vi "Generate Unique Header.vi"(8 "error in":errorcluster, 11 "mTEC Data in":refnum<class "mTEC Data.lvclass">) -> (0 "error out":errorcluster, 2 "Header":string[](array[string]), 3 "mTEC Data out":refnum<class "mTEC Data.lvclass">)   [LabVIEW 2014, in "Meerstetter Lib.lvlib" / "mTEC Data.lvclass"]
uses:
  mTEC Data.lvclass
  reusable/Data/Data.lvclass/Data.ctl
  reusable/Data/Read Data ID.vi
  reusable/Data/Data.lvclass
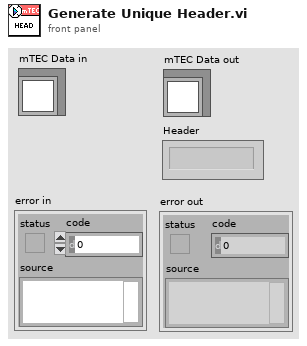
[diagram p1: front panel]
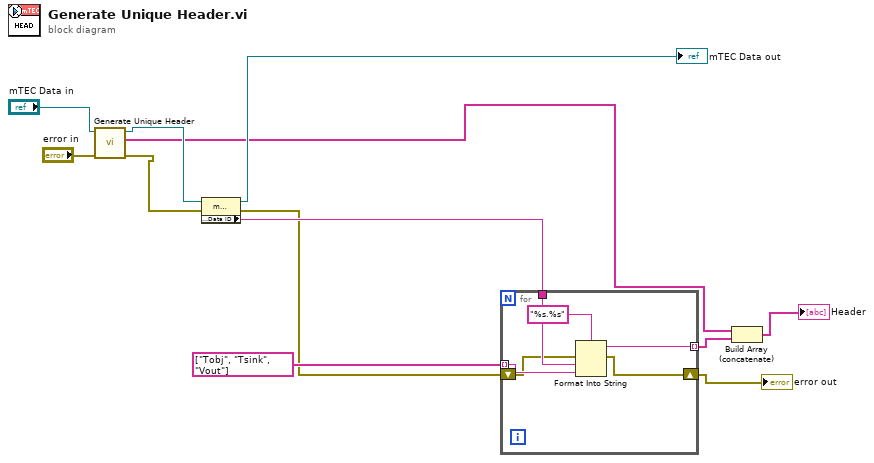
[diagram p0: block diagram]
diagram:
  n1 = call-parent "Generate Unique Header.vi"("error in"="error in", "Data in"="mTEC Data in") -> ("error out"=w8:errorcluster, "Header"=w2:string[], "Data out"=w9:refnum<class "mTEC Data.lvclass">)  [unwired: 7 in]
  n2 = property class="mTEC Data.lvclass"(reference=w9, error in=w8) -> (reference out=→"mTEC Data out":refnum<class "mTEC Data.lvclass">, error out=w6:errorcluster, "Accessors:Data ID"=w7:string)
  n3 = for {
    tunnel: string[] ["Tobj", "Tsink", "Vout"] -> [w17] mode=indexing
    tunnel: w7 -> [w18]
    tunnel: [w15] -> w3 mode=indexing
    shift-right: [w14] -> w4
    shift-left: w6 -> [w13]
    n4 = Format Into String(format string="%s.%s", error in=w13, w18, w17) -> (resulting string=w15:string, error out=w14:errorcluster)  [unwired: 1 in]
  }
  "error out" <- w4
  n5 = Build Array (concatenate)(w2, w3) -> (→"Header":string[])
